vi "Tosca-Validate Sequence Family.vi"(0 "Family in":T1, 5 "States":string[](array[string]), 7 "StimChans":cluster{string[]}[](array[cluster]), 9 "Params":cluster{"Parameter Names":string[]}[][](array[cluster]), 11 "error in (no error)":errorcluster) -> (4 "Family out":T1, 8 "errors":string, 10 "error":bool, 15 "error out":errorcluster)   [LabVIEW 2020]
uses:
  Typedefs/Tosca-Parameter Family.ctl
  Typedefs/Tosca-Parameter Table Element.ctl
  Typedefs/Tosca-Parameter Dimension.ctl
  Typedefs/Tosca-Family Order.ctl
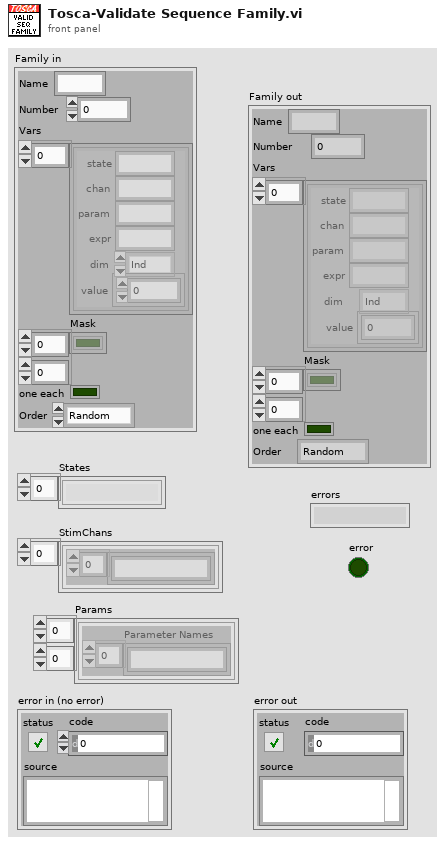
[diagram p1: front panel]
types:
  T1 = typedef "Tosca-Parameter Family.ctl" = cluster{"Name":string, "Number":i32, "Vars":T2[], "Mask":bool[][], "one each":bool, "Order":T4}
  T2 = typedef "Tosca-Parameter Table Element.ctl" = cluster{"state":string, "chan":string, "param":string, "expr":string, "dim":T3, "value":dbl[]}
  T3 = typedef "Tosca-Parameter Dimension.ctl" = enum16{"Ind", "X", "Y"}
  T4 = typedef "Tosca-Family Order.ctl" = enum16{"Random", "Sequential"}
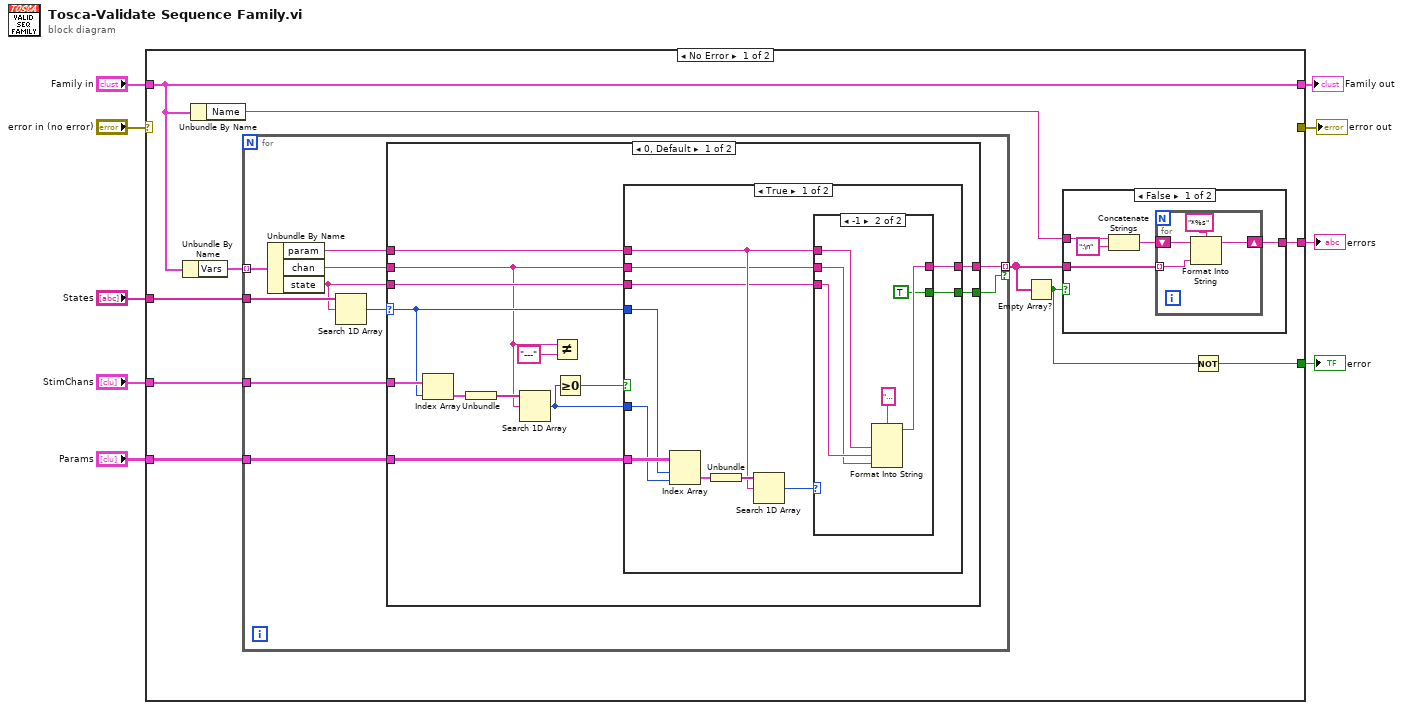
[diagram p0: block diagram]
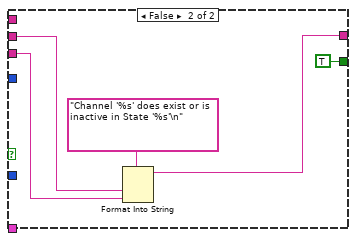
[diagram p4: hidden frame]
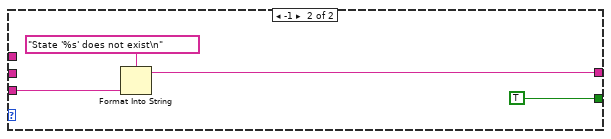
[diagram p5: hidden frame]
diagram:
  n1 = case shown="No Error" "error in (no error)" {
    selector: "error in (no error)" -> [_ w78]
    tunnel: "States" -> [w18 _]
    tunnel: "StimChans" -> [w17 _]
    tunnel: "Params" -> [w16 _]
    tunnel: "Family in" -> [w14 w79]
    tunnel: [w14 w79] -> w8
    tunnel: [_ w78] -> w3
    tunnel: [w12 _] -> w2
    tunnel: [w10 _] -> w1
    frame No Error {
      n2 = Unbundle By Name(w14) -> ("Vars"=w19:T2[])
      n3 = Unbundle By Name(w14) -> ("Name"=w13:string)
      n4 = for {
        tunnel: w19 -> [w38] mode=indexing
        tunnel: w18 -> [w37]
        tunnel: w17 -> [w35]
        tunnel: w16 -> [w31]
        tunnel: [w30] -> w15 mode=indexing if=w29
        n5 = Unbundle By Name(w38) -> ("param"=w32:string, "chan"=w33:string, "state"=w36:string)
        n6 = Search 1D Array(1D array=w37, element=w36) -> (index of element=w34:i32)  [unwired: 1 in]
        n7 = case shown="0, Default" w34 {
          selector: w34 -> [w47 _]
          tunnel: w36 -> [w45 w76]
          tunnel: w35 -> [w51 _]
          tunnel: w33 -> [w42 _]
          tunnel: w32 -> [w46 _]
          tunnel: w31 -> [w48 _]
          tunnel: [w44 w75] -> w30
          tunnel: [w43 TRUE] -> w29
          frame 0, Default {
            n8 = Index Array(array=w51, index=w47) -> (element=w50:cluster{string[]})
            n9 = Unbundle(w50) -> (w49:string[])
            n10 = Search 1D Array(1D array=w49, element=w42) -> (index of element=w40:i32)  [unwired: 1 in]
            n11 = Not Equal?(x=w42, y="---") -> ()  [unwired: 1 out]
            n12 = Greater Or Equal To 0?(x=w40) -> (x >= 0?=w39:bool)
            n13 = case shown="True" w39 {
              tunnel: w48 -> [w62 _]
              tunnel: w47 -> [w61 _]
              tunnel: w46 -> [w56 _]
              tunnel: w42 -> [w55 w72]
              tunnel: w45 -> [w54 w71]
              tunnel: [w53 w70] -> w44
              tunnel: [w52 TRUE] -> w43
              tunnel: w40 -> [w60 _]
              frame True {
                n14 = Index Array(array=w62, index (row)=w61, index (col)=w60) -> (element=w59:cluster{"Parameter Names":string[]})
                n15 = Unbundle(w59) -> ("Parameter Names"=w58:string[])
                n16 = Search 1D Array(1D array=w58, element=w56) -> (index of element=w57:i32)  [unwired: 1 in]
                n17 = case shown="-1" w57 {
                  tunnel: w56 -> [_ w67]
                  tunnel: w55 -> [_ w65]
                  tunnel: w54 -> [_ w66]
                  tunnel: [_ w64] -> w53
                  tunnel: [_ TRUE] -> w52
                  frame 0, Default {
                  }
                  frame -1 {
                    n18 = Format Into String(format string="Parameter '%s' is not valid for %s.%s\n", w67, w66, w65) -> (resulting string=w64:string)  [unwired: 2 in, 1 out]
                  }
                }
              }
              frame False {
                n19 = Format Into String(format string="Channel '%s' does exist or is inactive in State '%s'\n", w72, w71) -> (resulting string=w70:string)  [unwired: 2 in, 1 out]
              }
            }
          }
          frame -1 {
            n20 = Format Into String(format string="State '%s' does not exist\n", w76) -> (resulting string=w75:string)  [unwired: 2 in, 1 out]
          }
        }
      }
      n21 = Empty Array?(array=w15) -> (empty?=w11:bool)
      n22 = case shown="False" w11 {
        tunnel: w15 -> [w22 _]
        tunnel: w13 -> [w24 _]
        tunnel: [w20 _] -> w12
        frame False {
          n23 = Concatenate Strings(w24, ":\n" ("string")) -> (w21:string)
          n24 = for {
            tunnel: w22 -> [w25] mode=indexing
            shift-right: [w26] -> w20
            shift-left: w21 -> [w28]
            n25 = Format Into String(format string="*%s", initial string=w28, w25) -> (resulting string=w26:string)  [unwired: 1 in, 1 out]
          }
        }
        frame True {
        }
      }
      n26 = Not(x=w11) -> (.not. x?=w10:bool)
    }
    frame Error {
    }
  }
  "error out" <- w3
  "Family out" <- w8
  "errors" <- w2
  "error" <- w1
